vi "ble_write_by_service_characteristic_uint16.vi"(5 "Characteristic UUID":string, 6 "Connection Status":T1={"MAC Address"="", "cnx handle"=0, "cnx flags"=0, "Address Type"=125, "Connection Interval (ms)"=125, "Timeout(ms)"=125, "Latency"=0, "bonding handle"=0} {"Address Type" items=["Public", "Random"]}, 7 "Service UUID":string, 8 "error in (no error)":errorcluster, 9 "Value(16bit)":u16 format="%04x", 10 "Handle table":string[][](array[string]), 11 "COM Bluegiga in":refnum<visa-resource-name>) -> (0 "error out":errorcluster, 3 "COM Bluegiga out":refnum<visa-resource-name>)   [LabVIEW 2015]
uses:
  type_def/connection_status_bundle.ctl
  type_def/address_type.ctl
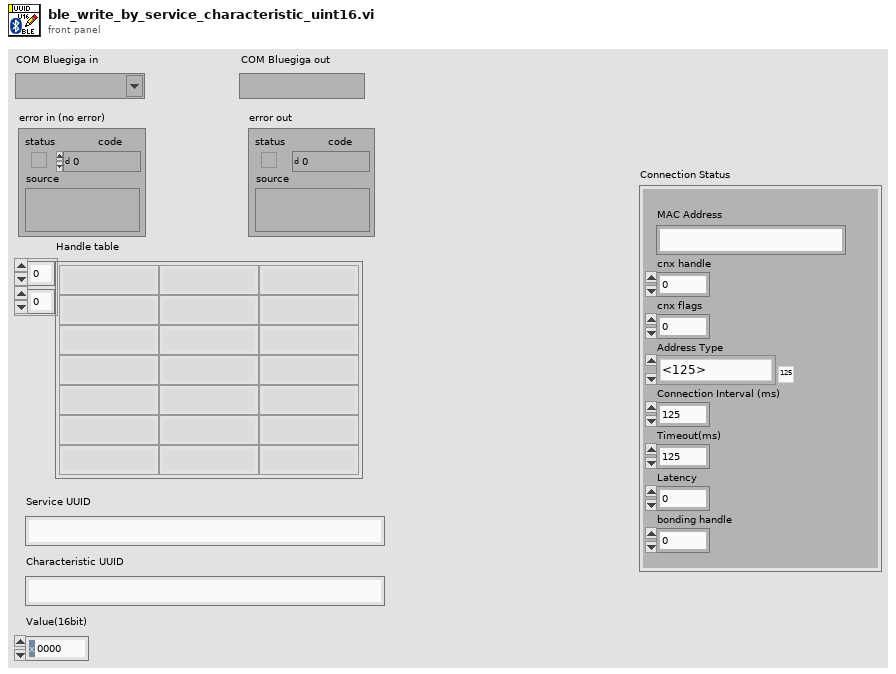
[diagram p1: front panel]
types:
  T1 = typedef "connection_status_bundle.ctl" = cluster{"MAC Address":string, "cnx handle":u8, "cnx flags":u8, "Address Type":T2, "Connection Interval (ms)":u16, "Timeout(ms)":u16, "Latency":u16, "bonding handle":u8}
  T2 = typedef "address_type.ctl" = u8
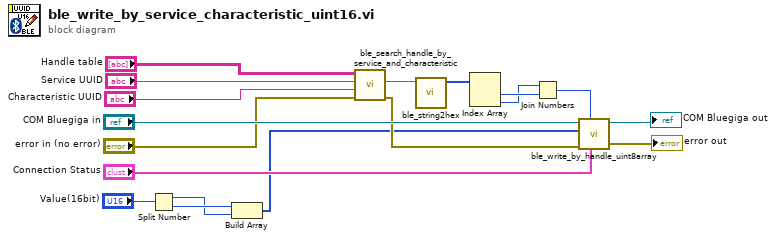
[diagram p0: block diagram]
diagram:
  n1 = Split Number(x="Value(16bit)") -> (hi(x)=w2:u8, lo(x)=w3:u8)
  n2 = Build Array(w3, w2) -> (w1:u8[])
  n3 = call "ble_search_handle_by_service_and_characteristic.vi"("error in (no error)"="error in (no error)", "Characteristic UUID"="Characteristic UUID", "Service UUID"="Service UUID", "Handle table"="Handle table") -> ("error out"=w7:errorcluster, "Handle"=w5:string)  [unwired: 6 in]
  n4 = call "ble_string2hex.vi"("HEX string IN"=w5) -> ("Byte Array IN (index0 LS byte)"=w6:u8[])  [unwired: 10 in]
  n5 = Index Array(array=w6) -> (element #1=w18:u8, element #2=w17:u8)  [unwired: 2 in]
  n6 = Join Numbers(hi=w17, lo=w18) -> ((hi.lo)=w16:u16)
  n7 = call "ble_write_by_handle_uint8array.vi"("Connection Status"="Connection Status", "Handle"=w16, "error in (no error)"=w7, "data (uint8array)"=w1, "COM Bluegiga in"="COM Bluegiga in") -> ("error out"=→"error out":errorcluster, "COM Bluegiga out"=→"COM Bluegiga out":refnum<visa-resource-name>)  [unwired: 5 in]
